vi "AuxNetwork.vi"   [LabVIEW 2020]
uses:
  AuxGlobals.vi
  <vilib>/Rock Robotics/Network Tables/NT Write Number.vi
  <vilib>/Rock Robotics/Network Tables/NT Write Boolean.vi
  <vilib>/Rock Robotics/Network Tables/NT Read Number.vi
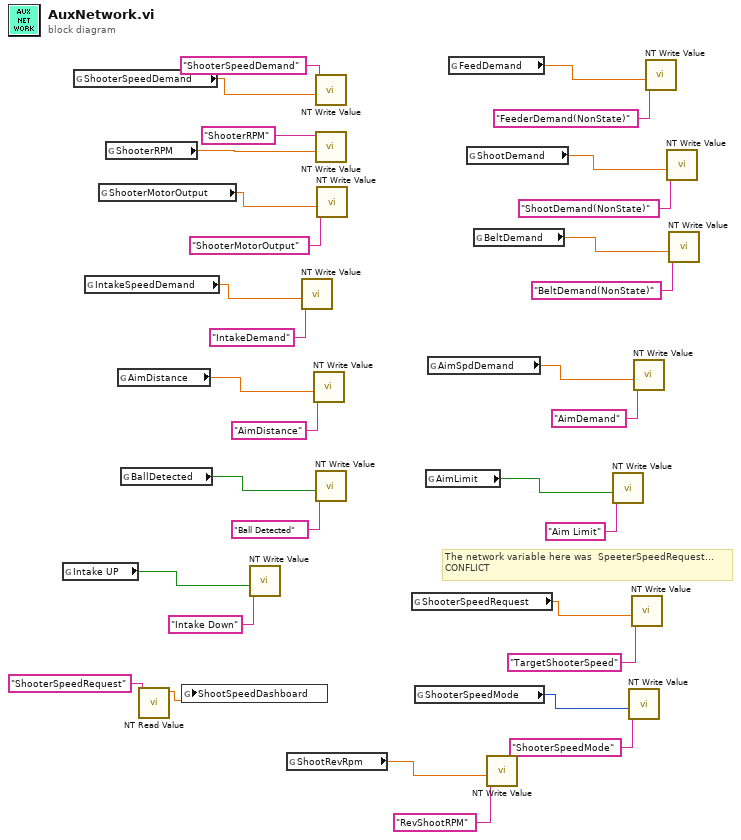
[diagram p0: block diagram]
diagram:
  # "The network variable here was  SpeeterSpeedRequest...\nCONFLICT"
  n1 = global read "AuxGlobals.vi" "Intake UP"() -> (w3:bool)
  n2 = global read "AuxGlobals.vi" "ShooterSpeedDemand"() -> (w27:dbl)
  n3 = global read "AuxGlobals.vi" "IntakeSpeedDemand"() -> (w21:dbl)
  n4 = global read "AuxGlobals.vi" "ShooterMotorOutput"() -> (w29:dbl)
  n5 = global read "AuxGlobals.vi" "ShooterRPM"() -> (w28:dbl)
  n6 = global read "AuxGlobals.vi" "AimDistance"() -> (w17:dbl)
  n7 = global read "AuxGlobals.vi" "BallDetected"() -> (w13:bool)
  n8 = call-poly <vilib>:"NT Read Value.vi"("Name"="ShooterSpeedRequest") -> ("Numeric"=w9:dbl)  [unwired: 9 in, 1 out]
  n9 = global write "AuxGlobals.vi" "ShootSpeedDashboard"(w9) -> ()
  n10 = call-poly <vilib>:"NT Write Value.vi"("Boolean"=w3, "Name"="Intake Down") -> ()  [unwired: 9 in, 1 out]
  n11 = global read "AuxGlobals.vi" "ShootRevRpm"() -> (w1:dbl)
  n12 = call-poly <vilib>:"NT Write Value.vi"("Numeric"=w21, "Name"="IntakeDemand") -> ()  [unwired: 9 in, 1 out]
  n13 = call-poly <vilib>:"NT Write Value.vi"("Numeric"=w17, "Name"="AimDistance") -> ()  [unwired: 9 in, 1 out]
  n14 = call-poly <vilib>:"NT Write Value.vi"("Numeric"=w27, "Name"="ShooterSpeedDemand") -> ()  [unwired: 9 in, 1 out]
  n15 = call-poly <vilib>:"NT Write Value.vi"("Numeric"=w28, "Name"="ShooterRPM") -> ()  [unwired: 9 in, 1 out]
  n16 = call-poly <vilib>:"NT Write Value.vi"("Boolean"=w13, "Name"="Ball Detected") -> ()  [unwired: 9 in, 1 out]
  n17 = call-poly <vilib>:"NT Write Value.vi"("Numeric"=w29, "Name"="ShooterMotorOutput") -> ()  [unwired: 9 in, 1 out]
  n18 = global read "AuxGlobals.vi" "ShooterSpeedRequest"() -> (w7:dbl)
  n19 = global read "AuxGlobals.vi" "ShooterSpeedMode"() -> (w5:i32)
  n20 = global read "AuxGlobals.vi" "AimLimit"() -> (w11:bool)
  n21 = global read "AuxGlobals.vi" "AimSpdDemand"() -> (w15:dbl)
  n22 = global read "AuxGlobals.vi" "FeedDemand"() -> (w23:dbl)
  n23 = global read "AuxGlobals.vi" "ShootDemand"() -> (w19:dbl)
  n24 = global read "AuxGlobals.vi" "BeltDemand"() -> (w25:dbl)
  n25 = call-poly <vilib>:"NT Write Value.vi"("Numeric"=w1, "Name"="RevShootRPM") -> ()  [unwired: 9 in, 1 out]
  n26 = call-poly <vilib>:"NT Write Value.vi"("Boolean"=w11, "Name"="Aim Limit") -> ()  [unwired: 9 in, 1 out]
  n27 = call-poly <vilib>:"NT Write Value.vi"("Numeric"=w5, "Name"="ShooterSpeedMode") -> ()  [unwired: 9 in, 1 out]
  n28 = call-poly <vilib>:"NT Write Value.vi"("Numeric"=w7, "Name"="TargetShooterSpeed") -> ()  [unwired: 9 in, 1 out]
  n29 = call-poly <vilib>:"NT Write Value.vi"("Numeric"=w15, "Name"="AimDemand") -> ()  [unwired: 9 in, 1 out]
  n30 = call-poly <vilib>:"NT Write Value.vi"("Numeric"=w23, "Name"="FeederDemand(NonState)") -> ()  [unwired: 9 in, 1 out]
  n31 = call-poly <vilib>:"NT Write Value.vi"("Numeric"=w19, "Name"="ShootDemand(NonState)") -> ()  [unwired: 9 in, 1 out]
  n32 = call-poly <vilib>:"NT Write Value.vi"("Numeric"=w25, "Name"="BeltDemand(NonState)") -> ()  [unwired: 9 in, 1 out]
